vi "Create FIFO.vi"(8 "error in (no error)":errorcluster, 9 "TX?":bool, 10 "FIFO Name":string, 11 "Comm FIFOs Virtual Folder":refnum<vi>) -> (0 "error out":errorcluster, 3 "Comm FIFOs Virtual Folder":refnum<vi>)   [LabVIEW 2014, in "SPI Engine Scripting.lvlib"]
doc: "Creates a FIFO in a specified project folder."
uses:
  SPI Engine Scripting.lvlib
  <vilib>/rvi/ClientSDK/Core/Script/Fifo/ProjectItem/Public/nirviPiFifoType_Size.ctl
  <vilib>/rvi/ClientSDK/Core/Script/Fifo/ProjectItem/Public/nirviPiFifoType_ArbitrationOption.ctl
  <vilib>/rvi/ClientSDK/Core/Script/Fifo/ProjectItem/Private/nirviPiFifo_OpenWithProjectItem.vi
  <vilib>/rvi/ClientSDK/Core/Script/Fifo/ProjectItem/Private/nirviPiFifo_SetDataType2.vi
  <vilib>/rvi/ClientSDK/Core/Script/Fifo/ProjectItem/Private/nirviPiFifo_SetSize.vi
  <vilib>/rvi/ClientSDK/Core/Script/Fifo/ProjectItem/Private/nirviPiFifo_SetArbitrationOptions.vi
  <vilib>/rvi/ClientSDK/Core/Script/Fifo/ProjectItem/Private/nirviPiFifo_CommitGlobal.vi
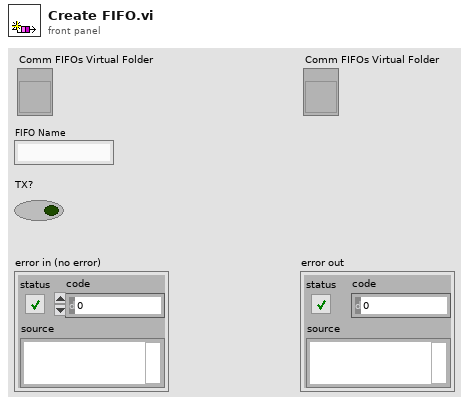
[diagram p1: front panel]
types:
  T1 = typedef "nirviPiFifoType_ArbitrationOption.ctl" = u16
  T2 = typedef "nirviPiFifoType_Size.ctl" = u32
  T3 = cluster{"Device ID":u8, "Data":u64, "Command":u8, "Node ID":u8, "Misc":u8}
  T4 = typedef "nirviPiFifo_State.ctl" = cluster{"Item":refnum<vi>, "Fifo":T5, "Dirty":bool, "XNode":refnum<vi>}
  T5 = typedef "niFpgaContainerState.ctl" = cluster{"displayName":string, "hardwareName":string, "dataType":T6, "elementTypeDescriptor":variant, "terminalTypeDescriptor":variant, "requestedNumberOfElements":u32, "memoryType":T7, "arbitrationForInterfaceA":T8, "numberOfElementsPerRead":u32, "arbitrationForInterfaceB":T8, "numberOfElementsPerWrite":u32, "VI_Defined":bool, "type":T9, "initializationParameters":T10, "disableOnOverflow/Underflow":bool, "interfaceConfiguration":T11, "controlLogic":T12, "actualNumberOfElements":u32, "dramSelection":string, "dramMaxOustandingRequests":i32, "dramIncludeByteEnables":bool, "dramGrantTime":u32, "fullEmulation":bool, "memoryInMultipleClockDomains":bool, "memoryLatency":T13}
  T6 = typedef "niFpgaDataTypeControl.ctl" = enum32{"Boolean", "I8", "I16", "I32", "I64", "U8", "U16", "U32", "U64", "FXP", "CustomControl", "SGL"}
  T7 = typedef "niFpgaContainerImplementationControl.ctl" = enum16{"Flip-Flops", "Look-Up Table", "Block Memory", "DRAM"}
  T8 = typedef "niFpgaContainerArbitrationOptionsControl.ctl" = enum16{"Always Arbitrate", "Arbitrate if Multiple Requestors Only", "Never Arbitrate"}
  T9 = typedef "niFpgaTransferTypeControl.ctl" = enum16{"Target-Scoped", "Host to Target - DMA", "Target to Host - DMA", "Peer to Peer Reader", "Peer to Peer Writer", "Bidirectional"}
  T10 = typedef "niFpgaContainerInitializationParameters.ctl" = cluster{"initialized":bool, "VI_Path":path, "initialData":variant}
  T11 = typedef "niFpgaMemoryInterfaceConfiguration.ctl" = enum16{"Read A-Write B", "Read A-Read B"}
  T12 = typedef "niFpgaFifoControlLogicControl.ctl" = enum16{"Slice Fabric", "Target Optimal", "Built-in"}
  T13 = typedef "niFpgaContainerMemoryLatencyControl.ctl" = u16
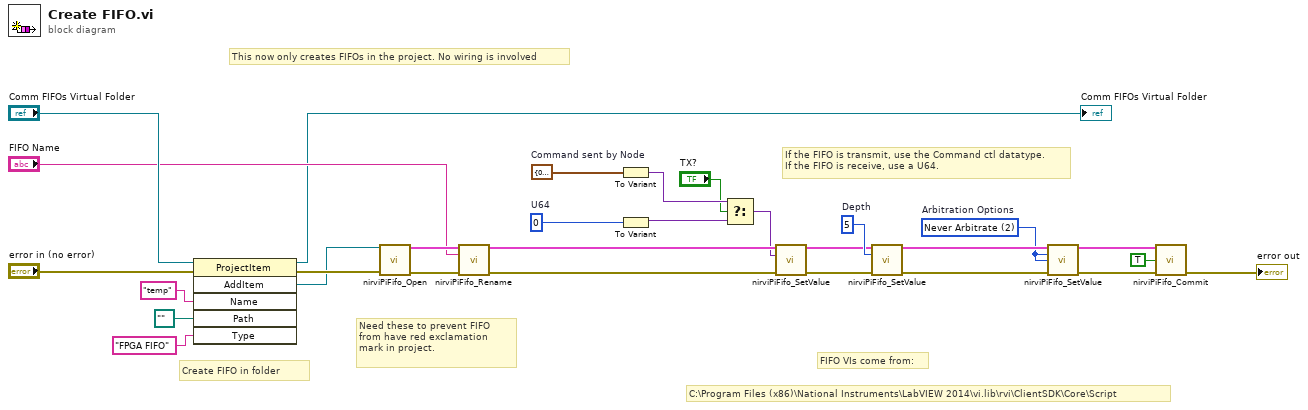
[diagram p0: block diagram]
diagram:
  w1 = T1 2 items=["Always Arbitrate", "Arbitrate if Multiple Accessors Only", "Never Arbitrate"]  # Arbitration Options
  w8 = T2 5  # Depth
  w13 = u64 0  # U64
  w14 = T3 {"Device ID"=0, "Data"=0, "Command"=0, "Node ID"=0, "Misc"=0}  # Command sent by Node
  # "If the FIFO is transmit, use the Command ctl datatype.\nIf the FIFO is receive, use a U64."
  # "FIFO VIs come from:"
  # "This now only creates FIFOs in the project. No wiring is involved"
  # "Create FIFO in folder"
  # "Need these to prevent FIFO from have red exclamation mark in project."
  # "C:\\Program Files (x86)\\National Instruments\\LabVIEW 2014\\vi.lib\\rvi\\ClientSDK\\Core\\Script"
  n1 = invoke class="ProjectItem" method="AddItem"(reference="Comm FIFOs Virtual Folder", error in="error in (no error)", "Name"="temp", "Path"=path "", "Type"="FPGA FIFO") -> (reference out=→"Comm FIFOs Virtual Folder":refnum<vi>, error out=w21:errorcluster, "AddItem"=w18:refnum<vi>)  [unwired: 1 in, 3 out]
  n2 = call-poly <vilib>:"nirviPiFifo_Open.vi"("Fifo Item"=w18, "error in (no error)"=w21) -> ("Reference"=w28:T4, "error out"=w29:errorcluster)  [unwired: 12 in]
  n3 = call <vilib>:"nirviPiFifo_Rename.vi"("reference"=w28, "name"="FIFO Name", "error in (no error)"=w29) -> ("reference"=w16:T4, "error out"=w15:errorcluster)  [unwired: 11 in]
  n4 = To Variant(anything=w14) -> (Variant=w12:variant)
  n5 = To Variant(anything=w13) -> (Variant=w10:variant)
  n6 = Select(t=w12, s="TX?", f=w10) -> (s? t:f=w9:variant)
  n7 = call-poly "nirviPiFifo_SetValue.vi"("Reference"=w16, "Data Type"=w9, "error in (no error)"=w15) -> ("Reference"=w6:T4, "error out"=w7:errorcluster)  [unwired: 11 in]
  n8 = call-poly "nirviPiFifo_SetValue.vi"("Reference"=w6, "Size"=w8, "error in (no error)"=w7) -> ("Reference"=w4:T4, "error out"=w5:errorcluster)  [unwired: 11 in]
  n9 = call-poly "nirviPiFifo_SetValue.vi"("Reference"=w4, "Read Arbitration"=w1, "Write Arbitration"=w1, "error in (no error)"=w5) -> ("Reference"=w2:T4, "error out"=w3:errorcluster)  [unwired: 10 in]
  n10 = call-poly <vilib>:"nirviPiFifo_Commit.vi"("Reference"=w2, "Close Reference?"=TRUE, "error in (no error)"=w3) -> ("error out"=→"error out":errorcluster)  [unwired: 11 in, 1 out]
